vi "Facade.vi"(0 "Data In":T4, 2 "Display State In":T2, 3 "Container State":T3) -> (6 "Data Out":T4, 7 "Display State Out":T2, 8 "Action":T1)   [LabVIEW 2017, in "XListGraph.lvlib" / "XListGraph.xctl"]
uses:
  XListGraph.xctl
  Data.ctl
  <vilib>/_xctls/Container State.ctl
  State.ctl
  Support/def-XListGraphOper.ctl
  <vilib>/_xctls/Action.ctl
  <userlib>/_OpenG.lib/array/array.llb/Index 1D Array Elements (String)__ogtk.vi
  <userlib>/_OpenG.lib/array/array.llb/Filter 1D Array (String)__ogtk.vi
  <userlib>/_OpenG.lib/string/string.llb/Trim Whitespace (String Array)__ogtk.vi
  <userlib>/_OpenG.lib/array/array.llb/Filter 1D Array with Scalar (I32)__ogtk.vi
  <userlib>/_OpenG.lib/array/array.llb/Filter 1D Array (I32)__ogtk.vi
  <userlib>/_OpenG.lib/array/array.llb/Remove Duplicates from 1D Array (I32)__ogtk.vi
  <userlib>/_OpenG.lib/array/array.llb/Sort 1D Array (I32)__ogtk.vi
  <userlib>/_OpenG.lib/array/array.llb/Search 1D Array (String)__ogtk.vi
  <vilib>/_xctls/XControlSupport.lvlib
panel:
  in  "Listbox":i32[](listbox)
  out "Waveform Graph":waveform(dbl)[](graph)
  in  "Tab":enum32{""}(tab)
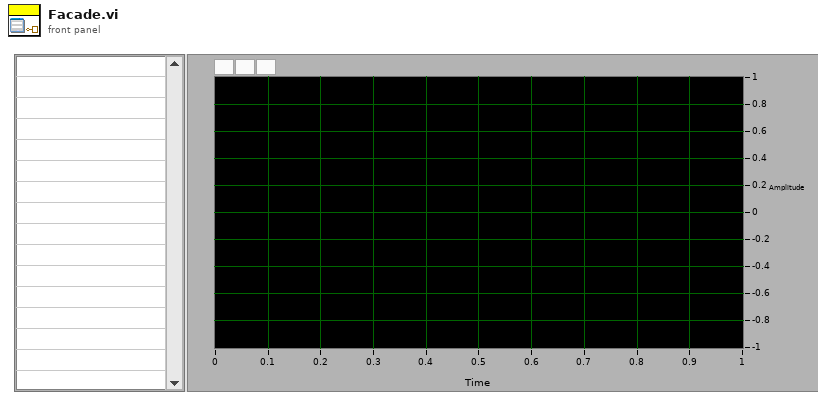
[diagram p1: front panel]
types:
  T1 = typedef "XControlSupport.lvlib/Action.ctl" = cluster{"Data Changed?":bool, "State Changed?":bool, "Action Name":string}
  T2 = typedef "XListGraph.lvlib/XListGraph.xctl/State.ctl" = cluster{"ListWindowSpliterPos":i32, "ListWindowSpliterLocked":bool, "axes":cluster{"X":cluster{"Label":string, "Unit":string}, "Y":cluster{"Label":string, "Unit":string}}, "Next State":string, "User Event":refnum<user-event>, "Plot Names":string[], "Visible Plot Names":string[], "Selected Plot Names":string[]}
  T3 = typedef "XControlSupport.lvlib/Container State.ctl" = cluster{"Indicator?":bool, "Run Mode?":bool, " Refnum":refnum<vi>}
  T4 = typedef "XListGraph.lvlib/XListGraph.xctl/Data.ctl" = waveform(dbl)[]
  T5 = typedef "LVPoint32TypeDef.ctl" = cluster{"Horizontal":i32, "Vertical":i32}
  T6 = typedef "LVRectTypeDef.ctl" = cluster{"Left":i16, "Top":i16, "Right":i16, "Bottom":i16}
  T7 = cluster{"Core":cluster{"Current VI Reference":refnum<vi>, "Close Panel on Exit?":bool}, "Splitter":refnum<vi>, "GraphRef":refnum<vi>, "ListboxRef":refnum<vi>, "Tab":refnum<vi>, "Active Menu Items":string[]}
  T8 = cluster{"Current VI Reference":refnum<vi>, "Close Panel on Exit?":bool}
  T9 = typedef "XListGraph.lvlib/XListGraph.xctl/def-wfProps.ctl" = cluster{"NI_ChannelName":string, "NI_ChannelUnit":string}
  T10 = typedef "XListGraph.lvlib/XListGraph.xctl/def-XListGraphOper.ctl" = u16
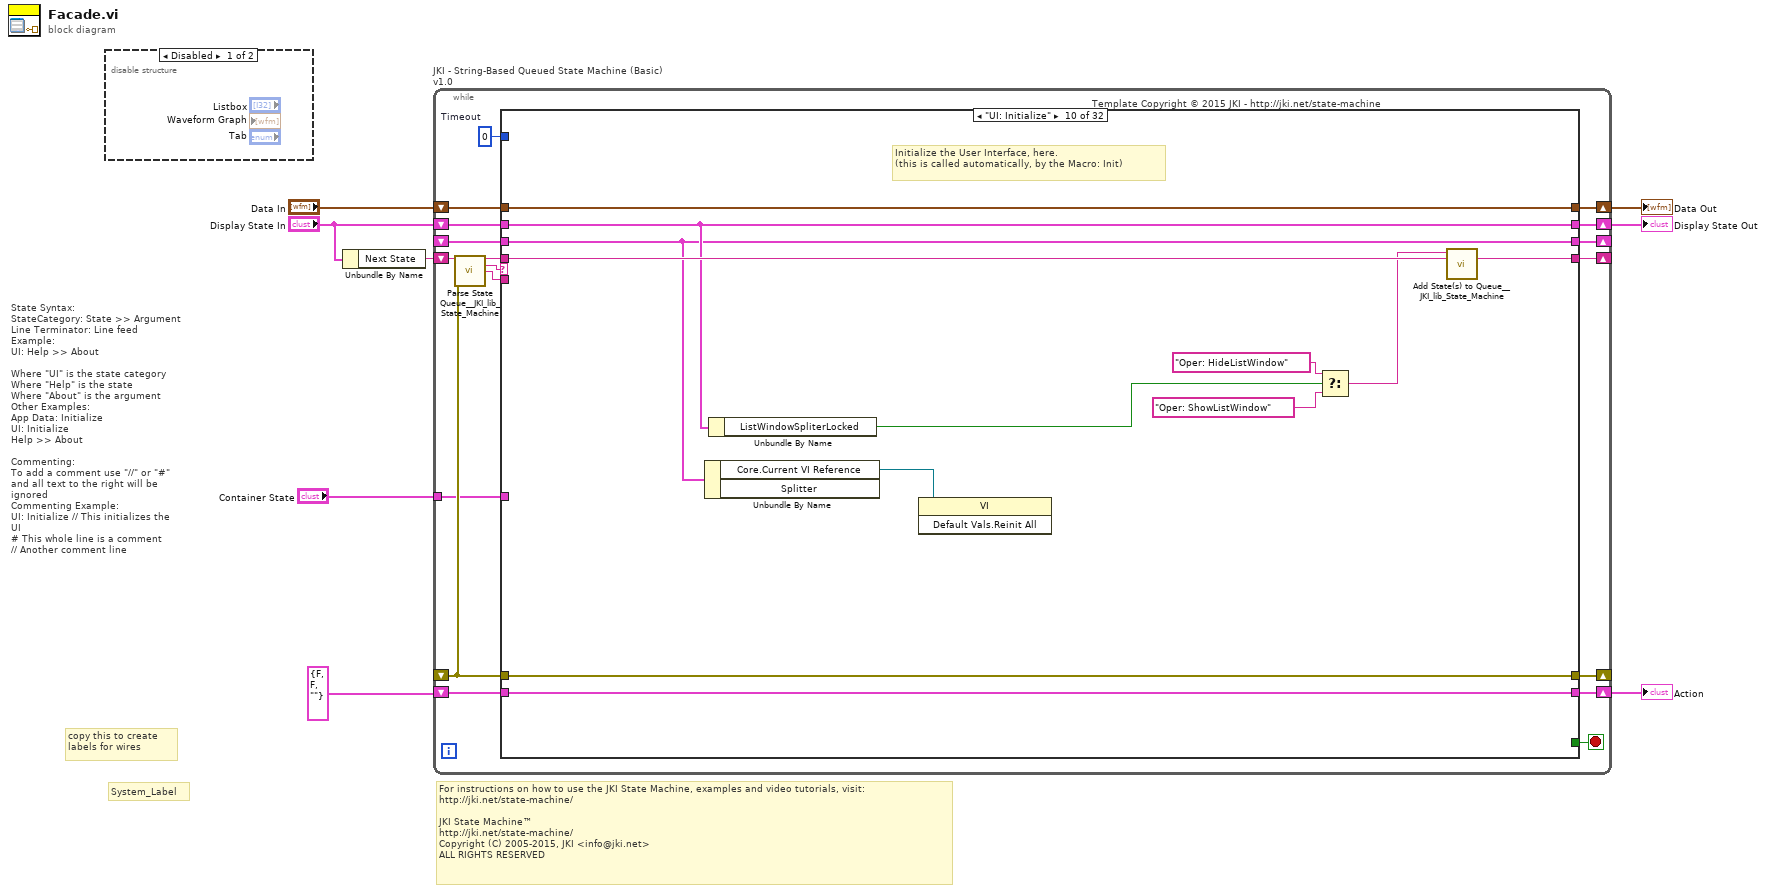
[diagram p0: block diagram]
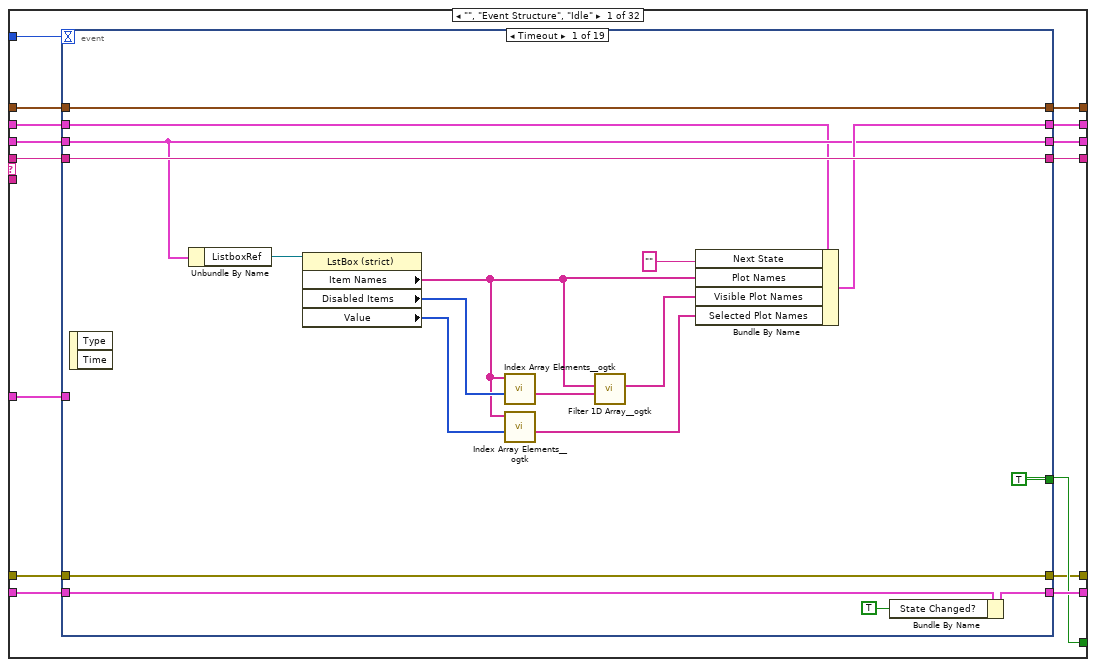
[diagram p3: hidden frame]
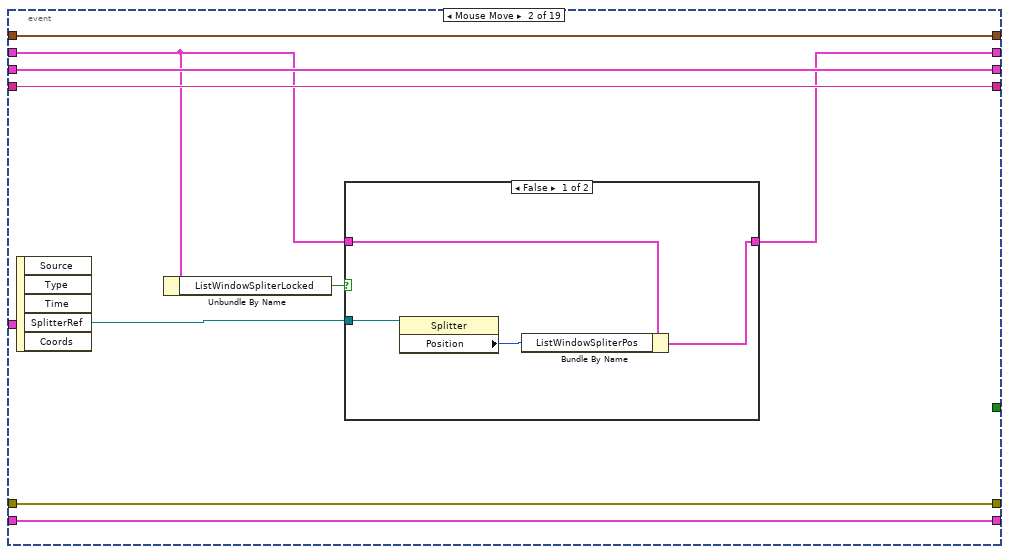
[diagram p4: hidden frame]
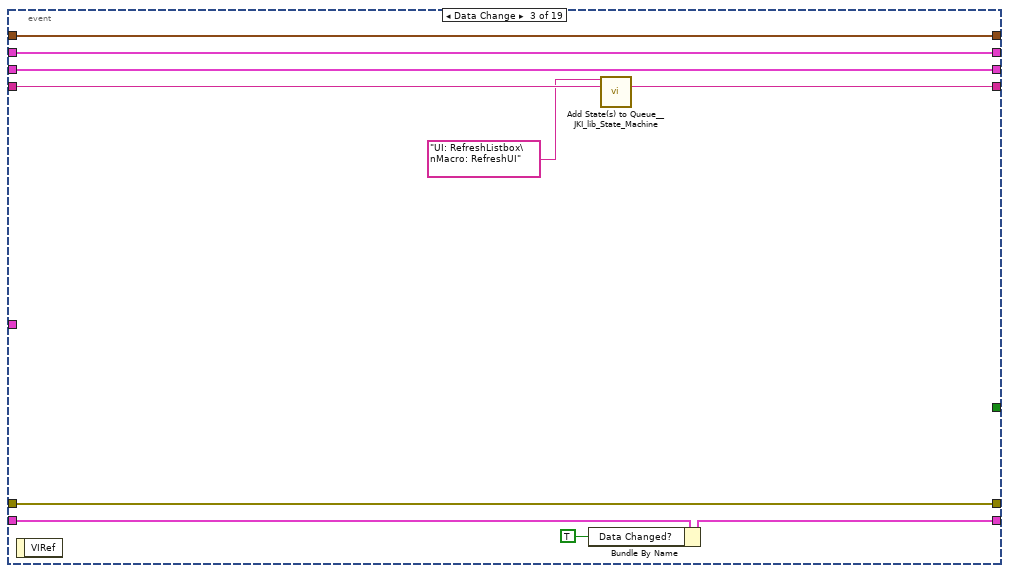
[diagram p6: hidden frame]
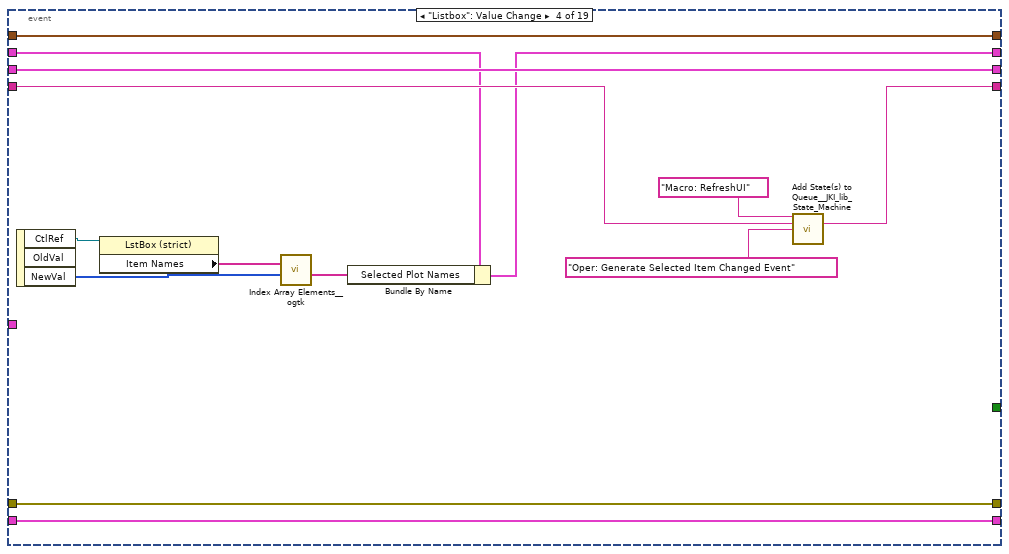
[diagram p7: hidden frame]
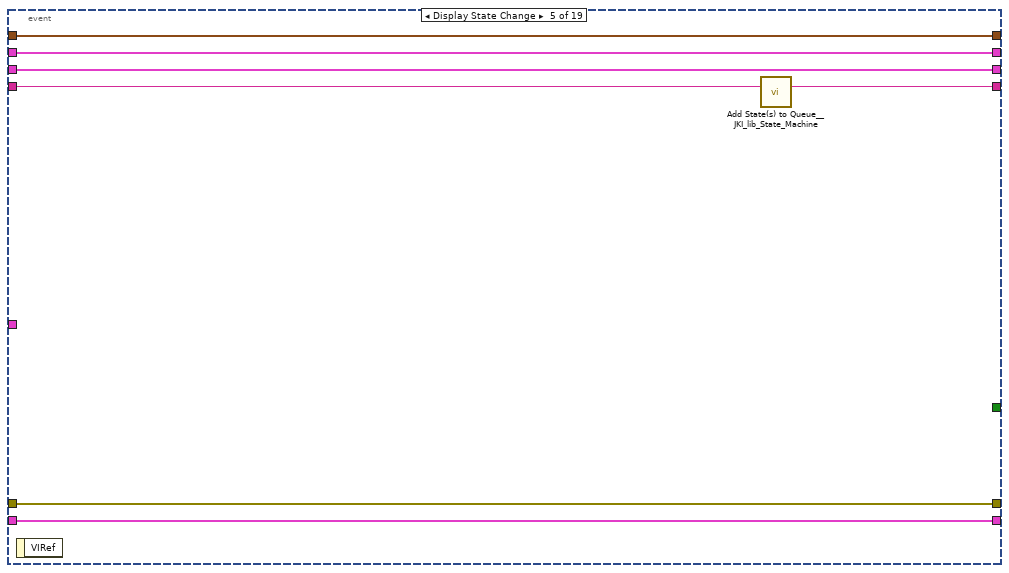
[diagram p8: hidden frame]
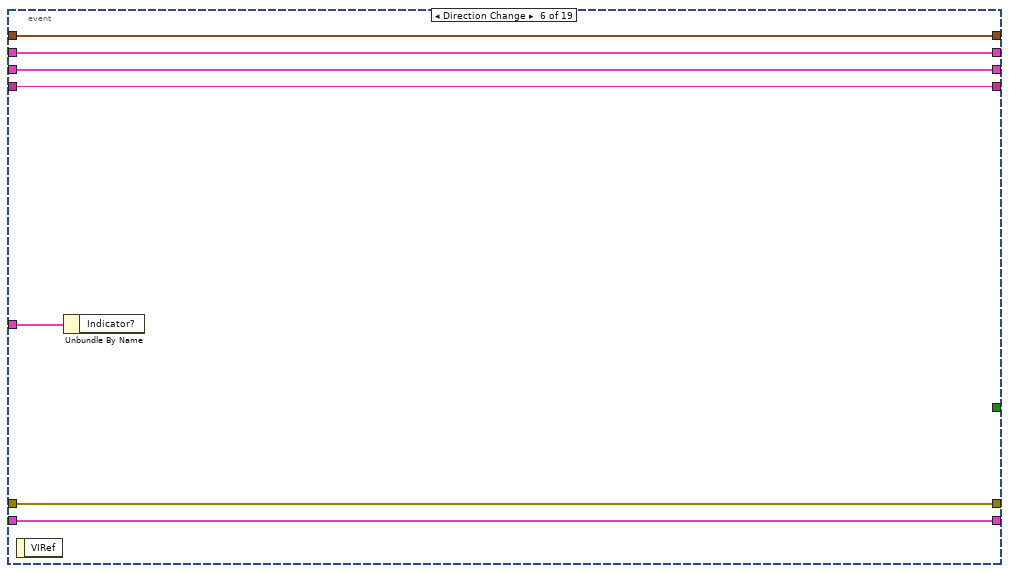
[diagram p9: hidden frame]
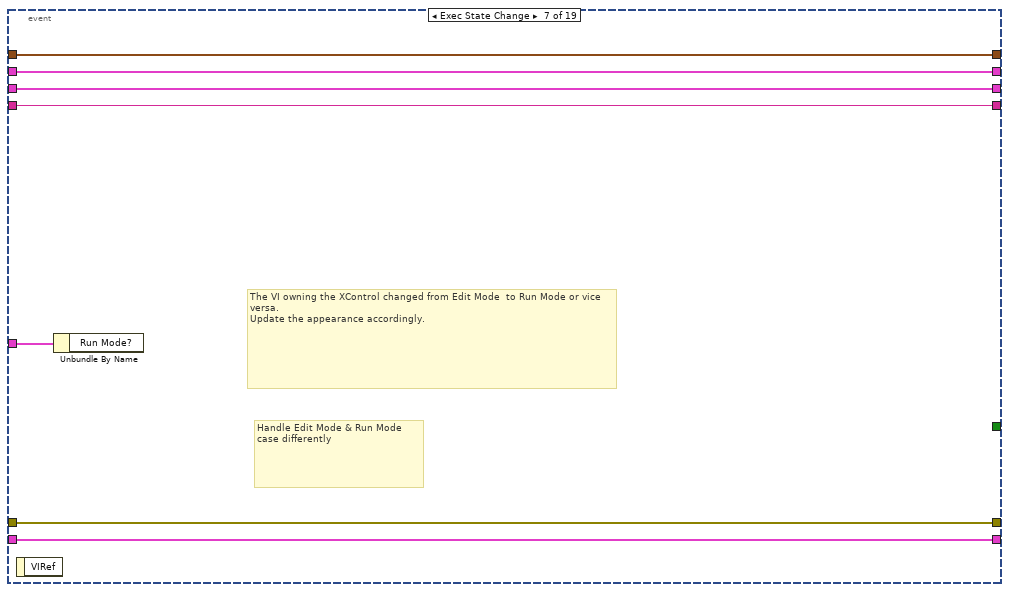
[diagram p10: hidden frame]
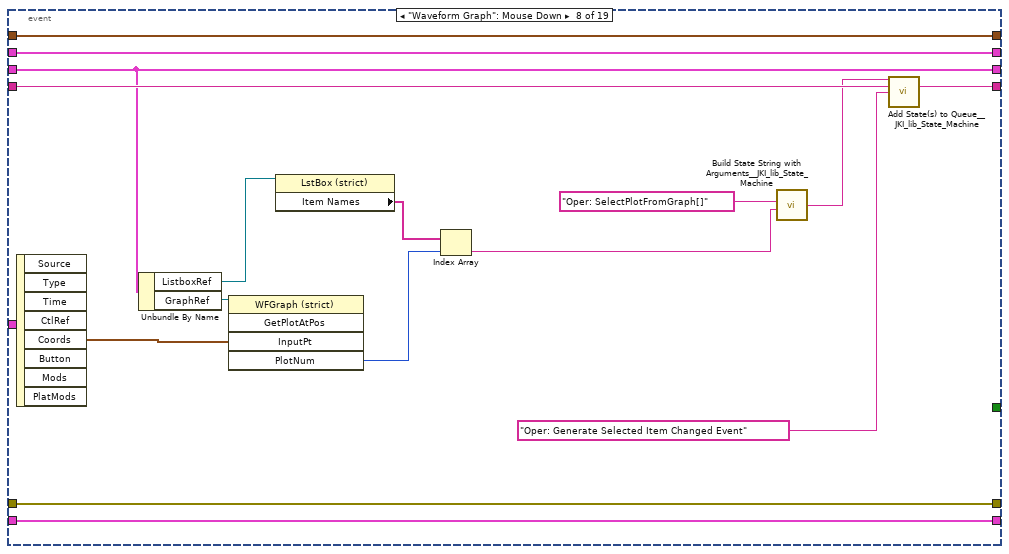
[diagram p11: hidden frame]
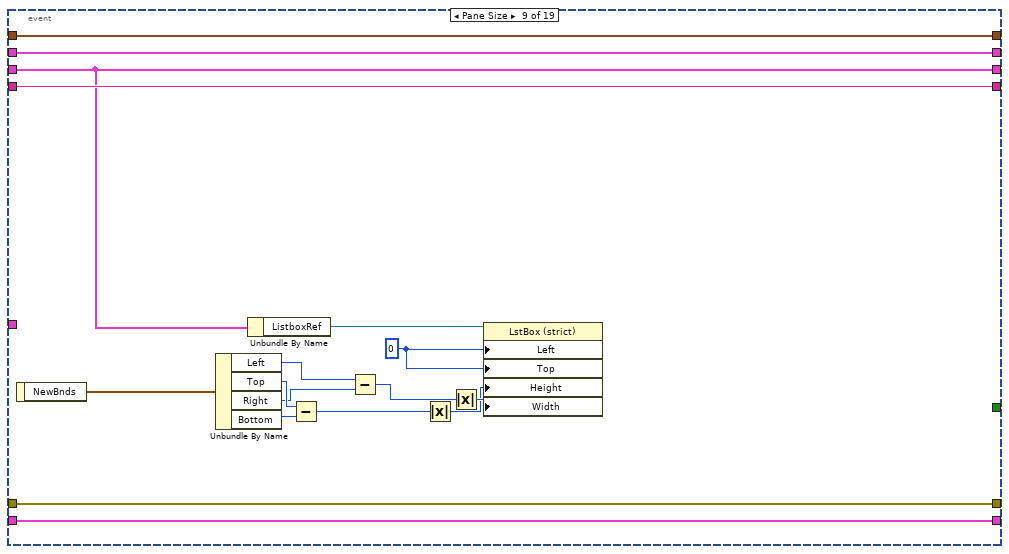
[diagram p12: hidden frame]
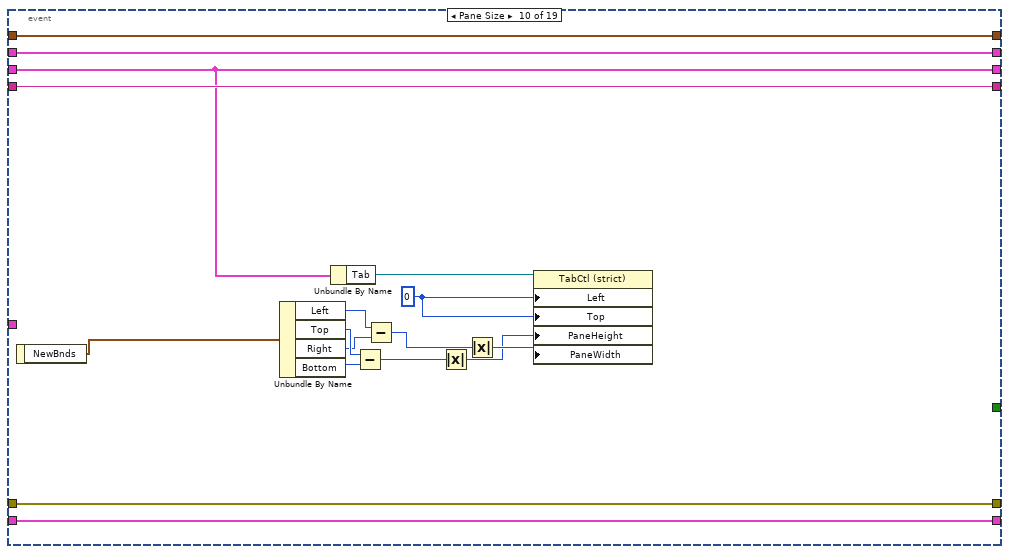
[diagram p13: hidden frame]
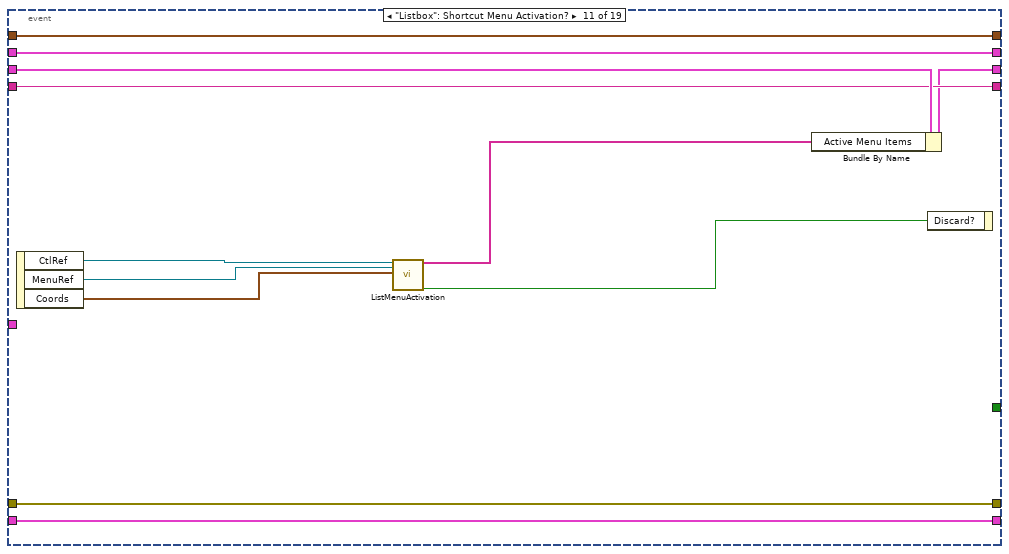
[diagram p14: hidden frame]
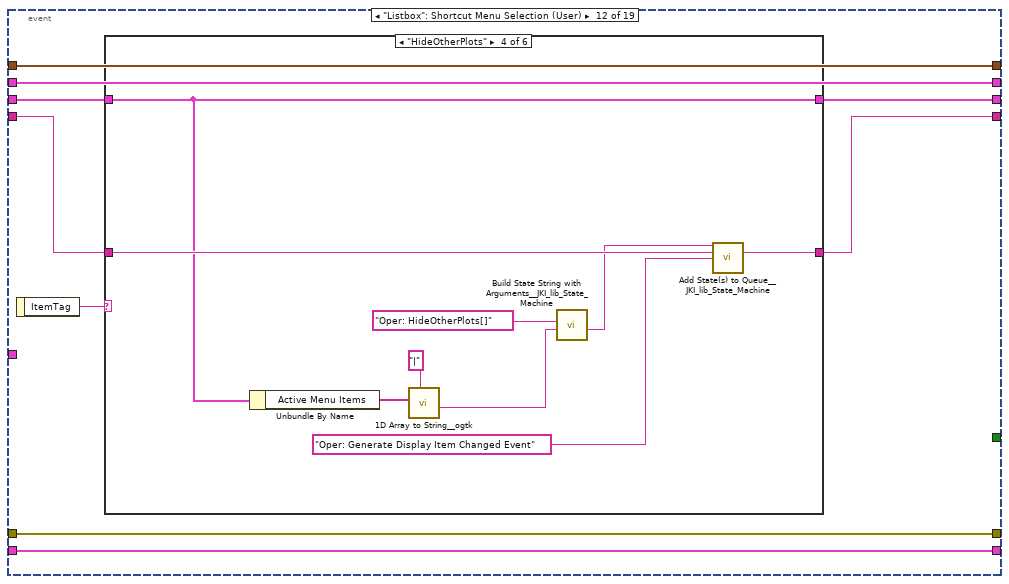
[diagram p15: hidden frame]
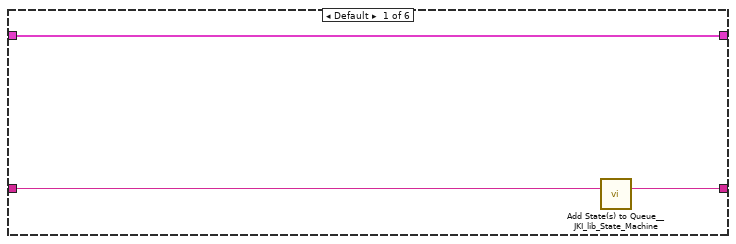
[diagram p16: hidden frame]
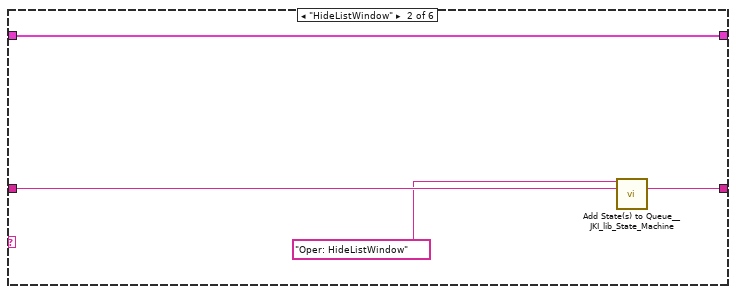
[diagram p17: hidden frame]
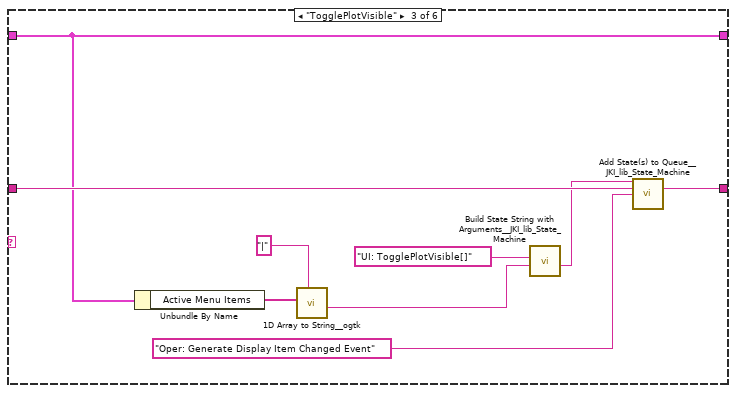
[diagram p18: hidden frame]
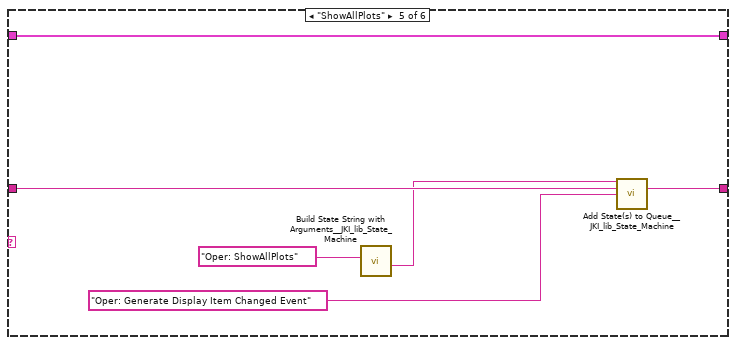
[diagram p19: hidden frame]
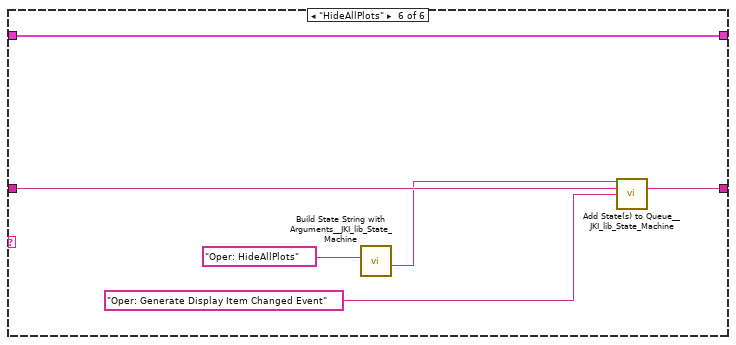
[diagram p20: hidden frame]
diagram:
  # "For instructions on how to use the JKI State Machine, examples and video tutorials, visit:\nhttp://jki.net/state-machine/\n\nJKI State Machine™\nhttp://jki.net/state-machine/\nCopyright (C) 2005-2015, JKI <info@jki.net>\nALL RIGHTS RESERVED"
  # "State Syntax:\nStateCategory: State >> Argument\nLine Terminator: Line feed\nExample:\nUI: Help >> About\n\nWhere \"UI\" is the state category\nWhere \"Help\" is the state\nWhere \"About\" is the argument\nOther Examples:\nApp Data: Initialize\nUI: Initialize\nHelp >> About\n\nCommenting:\nTo add a comment use \"//\" or \"#\" and all text to the right will be ignored\nCommenting Example:\nUI: Initialize // This initializes the UI\n# This whole line is a comment\n// Another comment line"
  # "copy this to create labels for wires"
  # "System_Label"
  n1 = disable-structure shown="Disabled" {
    frame Disabled {
    }
    frame Enabled {
    }
  }
  n2 = Unbundle By Name("Display State In") -> ("Next State"=w1:string)
  n3 = while "JKI - String-Based Queued State Machine (Basic) v1.0" {
    shift-right: [w19] -> _
    shift-left: _ -> [w18]
    shift-right: [w22] -> _
    shift-left: _ -> [w16]
    shift-right: [w21] -> _
    shift-left: w1 -> [w23]
    shift-right: [w14] -> w7
    shift-left: T1 {"Data Changed?"=FALSE, "State Changed?"=FALSE, "Action Name"=""} ("Action") -> [w15]
    shift-right: [w11] -> w4
    shift-left: "Data In" -> [w13]
    shift-right: [w10] -> w5
    shift-left: "Display State In" -> [w12]
    tunnel: "Container State" -> [w9]
    stop <- w20 stop-if-true
    w17 = 0  # Timeout
    # "Template Copyright © 2015 JKI - http://jki.net/state-machine"
    n4 = call <vilib>:"Parse State Queue__JKI_lib_State_Machine.vi"("State Queue"=w23, "Error In (no error)"=w16) -> ("Remaining States"=w25:string, "Current State"=w26:string, "Arguments"=w24:string)  [unwired: 11 in]
    n5 = case shown="\"UI: Initialize\"" w26 {
      selector: w26 -> [_ _ w304 _ _ _ _ _ _ _ _ _ _ _ _ _ _ _ _ _ _ _ _ _ _ _ _ _ _ _ _ _]
      tunnel: w25 -> [w27 w300 w308 w323 w332 w339 w352 w361 w368 w380 w389 w398 w411 w451 w467 w487 w510 w518 w526 w533 w538 w550 w569 w589 w605 w625 w635 w667 w677 w687 w699 w707]
      tunnel: w24 -> [_ _ _ _ _ _ _ _ _ _ w384 _ _ _ _ w476 _ _ _ _ _ _ w567 w587 w603 w623 w634 w655 _ _ _ _]
      tunnel: w18 -> [w29 w297 w306 w319 w329 w336 _ w356 w365 w374 w387 w394 w403 w426 w461 w481 w507 w515 w523 w530 w534 w544 w565 w586 w602 w622 w643 w654 w674 w681 w694 w702]
      tunnel: [w32 w298 w310 w320 errorcluster {"status"=FALSE, "code"=0, "source"=""} ("error out") w337 w349 w357 w366 w378 w385 w397 w412 w452 w466 w492 w508 w516 w524 w531 w543 w555 w574 w594 w610 w630 w651 w665 w678 w688 w700 w708] -> w22
      tunnel: w16 -> [w31 w298 w309 w320 w328 w337 w349 w358 w366 w378 w386 w397 w412 w452 w466 w492 w508 w516 w524 w531 w543 w555 w574 w594 w610 w630 w651 w665 w678 w688 w700 w708]
      tunnel: [w28 w299 w307 w322 w331 w338 w351 w360 w367 w379 w388 w398 w411 w451 w467 w488 w509 w517 w525 w532 w539 w551 w570 w590 w606 w626 w647 w666 w677 w687 w699 w707] -> w21
      tunnel: [w33 _ _ _ _ _ _ _ _ _ _ _ _ _ _ _ _ _ _ _ _ _ _ _ _ _ _ _ _ _ _ _] -> w20
      tunnel: [w30 w297 w306 w321 w329 w336 w350 w356 w365 w374 w387 w394 w403 w426 w461 w481 w507 w515 w523 w530 w534 w544 w565 w586 w602 w622 w643 w654 w674 w681 w694 w702] -> w19
      tunnel: w17 -> [w41 _ _ _ _ _ _ _ _ _ _ _ _ _ _ _ _ _ _ _ _ _ _ _ _ _ _ _ _ _ _ _]
      tunnel: w15 -> [w38 w296 w303 w317 w326 w335 w347 w355 w364 w377 w383 w400 w410 w450 w469 w491 w506 w513 w521 w529 w542 w554 w573 w593 w609 w629 w650 w664 w676 w686 w698 w706]
      tunnel: [w37 w296 w303 w317 w326 w335 w347 w355 w364 w377 w383 w400 w410 w450 w469 w491 w506 w513 w521 w529 w542 w554 w573 w593 w609 w629 w650 w664 w676 w686 w698 w706] -> w14
      tunnel: w13 -> [w40 w295 w302 w316 w325 w334 w346 w354 w363 w376 w382 w395 w408 w438 w463 w490 w505 w512 w520 w528 w541 w553 w572 w592 w608 w628 w649 w663 w675 w685 w697 w705]
      tunnel: w12 -> [w36 w294 w301 w315 w324 w333 w345 w353 w362 w375 w381 w399 w402 w447 w468 w489 w504 w511 w519 w527 w540 w552 w571 w591 w607 w627 w648 w662 w673 w684 w693 w701]
      tunnel: [w39 w295 w302 w316 w325 w334 w346 w354 w363 w376 w382 w395 w408 w438 w463 w490 w505 w512 w520 w528 w541 w553 w572 w592 w608 w628 w649 w663 w675 w685 w697 w705] -> w11
      tunnel: [w35 w294 w301 w315 w324 w333 w345 w353 w362 w375 w381 w399 w402 w447 w468 w489 w504 w511 w519 w527 w540 w552 w571 w591 w607 w627 w648 w662 w669 w683 w693 w701] -> w10
      tunnel: w9 -> [w34 _ _ _ _ _ _ _ _ _ _ _ _ _ _ _ _ _ _ _ _ _ _ _ _ _ _ _ _ _ _ _]
      frame "", "Event Structure", "Idle" {
        n6 = event shown="[0] Timeout" {
          selector: _ -> [_ _ _ _ _ _ _ _ _ _ _ _ _ _ _ _ _ _ _]
          dyn-events: _ -> [_ _ _ _ _ _ _ _ _ _ _ _ _ _ _ _ _ _ _]
          timeout: w41 -> [_ _ _ _ _ _ _ _ _ _ _ _ _ _ _ _ _ _ _]
          tunnel: w36 -> [w42 w61 w83 w85 w98 w110 w117 w134 w151 w168 w180 w189 w232 w239 w246 w248 w261 w276 w293]
          tunnel: [w54 w62 w83 w84 w98 w110 w117 w134 w151 w168 w180 w189 w232 w239 w246 w248 w261 w276 w293] -> w35
          tunnel: [TRUE _ _ _ _ _ _ _ _ _ _ _ _ _ _ _ _ _ _] -> w33
          tunnel: w34 -> [_ _ _ _ _ w111 w118 _ _ _ _ _ _ _ _ _ _ _ _]
          tunnel: w40 -> [w57 w68 w77 w95 w104 w109 w116 w133 w150 w167 w179 w188 w231 w238 w245 w253 w260 w275 w292]
          tunnel: [w57 w68 w77 w95 w104 w109 w116 w133 w150 w167 w179 w188 w231 w238 w245 w253 w260 w275 w292] -> w39
          tunnel: [w52 w67 w81 w97 w103 w108 w115 w132 w149 w166 w178 w187 w230 w237 w244 w252 w259 w274 w291] -> w37
          tunnel: w38 -> [w58 w67 w82 w97 w103 w108 w115 w132 w149 w166 w178 w187 w230 w237 w244 w252 w259 w274 w291]
          tunnel: [w56 w66 w79 w96 w102 w107 w114 w131 w137 w165 w174 w185 w229 w236 w243 w251 w258 w273 w290] -> w32
          tunnel: w31 -> [w56 w66 w79 w96 w102 w107 w114 w131 w137 w165 w174 w185 w229 w236 w243 w251 w258 w273 w290]
          tunnel: [w50 w65 w78 w91 w101 w106 w113 w126 w135 w152 w175 w182 w228 w235 w242 w250 w257 w272 w289] -> w30
          tunnel: w29 -> [w50 w65 w78 w91 w101 w106 w113 w126 w135 w152 w177 w181 w228 w235 w242 w250 w257 w272 w289]
          tunnel: [w55 w64 w76 w94 w100 w105 w112 w128 w136 w164 w176 w183 w227 w234 w241 w249 w254 w271 w285] -> w28
          tunnel: w27 -> [w55 w64 w75 w93 w99 w105 w112 w127 w136 w164 w176 w184 w227 w234 w241 w249 w255 w271 w284]
          event Timeout {
            n7 = event-data() -> ()  [unwired: 1 in, 2 out]
            n8 = Unbundle By Name(w50) -> ("ListboxRef"=w49:refnum<vi>)
            n9 = property class="LstBox (strict)"(reference=w49) -> ("Item Names"=w45:string[], "Disabled Items"=w48:i32[], "Value"=w44:i32[])  [unwired: 1 in, 2 out]
            n10 = call-poly <userlib>:"Index Array Elements__ogtk.vi"("indices"=w48, "array"=w45) -> ("elements"=w47:string[])  [unwired: 9 in]
            n11 = call-poly <userlib>:"Index Array Elements__ogtk.vi"("indices"=w44, "array"=w45) -> ("elements"=w43:string[])  [unwired: 9 in]
            n12 = call-poly <userlib>:"Filter 1D Array__ogtk.vi"("items to filter"=w47, "array"=w45) -> ("filtered array"=w46:string[])  [unwired: 4 in, 1 out]
            n13 = Bundle By Name(cluster=w42, "Next State"="", "Plot Names"=w45, "Visible Plot Names"=w46, "Selected Plot Names"=w43) -> (w54:T2)
            n14 = Bundle By Name(cluster=w58, "State Changed?"=TRUE) -> (w52:T1)
          }
          event Mouse Move {
            n15 = event-data() -> ("SplitterRef"=w63:refnum<vi>)  [unwired: 1 in, 4 out]
            n16 = Unbundle By Name(w61) -> ("ListWindowSpliterLocked"=w60:bool)
            n17 = case shown="False" w60 {
              tunnel: w63 -> [w72 _]
              tunnel: [w71 w73] -> w62
              tunnel: w61 -> [w69 w73]
              frame False {
                n18 = property class="Splitter"(reference=w72) -> ("Position"=w70:i32)  [unwired: 1 in, 2 out]
                n19 = Bundle By Name(cluster=w69, "ListWindowSpliterPos"=w70) -> (w71:T2)
              }
              frame True {
              }
            }
          }
          event Data Change {
            n20 = event-data() -> ()  [unwired: 1 in, 1 out]
            n21 = Bundle By Name(cluster=w82, "Data Changed?"=TRUE) -> (w81:T1)
            n22 = call <vilib>:"Add State(s) to Queue__JKI_lib_State_Machine.vi"("State(s) in Front (\"\")"="UI: RefreshListbox\nMacro: RefreshUI" ("State(s) in Front (\"\")"), "State(s) in (\"\")"=w75) -> ("States Out"=w76:string)  [unwired: 13 in]
          }
          event "Listbox": Value Change {
            n23 = event-data() -> ("CtlRef"=w88:refnum<vi>, "NewVal"=w89:i32[])  [unwired: 1 in, 1 out]
            n24 = property class="LstBox (strict)"(reference=w88) -> ("Item Names"=w87:string[])  [unwired: 1 in, 2 out]
            n25 = call-poly <userlib>:"Index Array Elements__ogtk.vi"("indices"=w89, "array"=w87) -> ("elements"=w86:string[])  [unwired: 9 in]
            n26 = Bundle By Name(cluster=w85, "Selected Plot Names"=w86) -> (w84:T2)
            n27 = call <vilib>:"Add State(s) to Queue__JKI_lib_State_Machine.vi"("State(s) in Front (\"\")"="Macro: RefreshUI" ("State(s) in Front (\"\")"), "State(s) in (\"\")"=w93, "State(s) at Back (\"\")"="Oper: Generate Selected Item Changed Event" ("State(s) at Back (\"\")")) -> ("States Out"=w94:string)  [unwired: 12 in]
          }
          event Display State Change {
            n28 = event-data() -> ()  [unwired: 1 in, 1 out]
            n29 = call <vilib>:"Add State(s) to Queue__JKI_lib_State_Machine.vi"("State(s) in (\"\")"=w99) -> ("States Out"=w100:string)  [unwired: 14 in]
          }
          event Direction Change {
            n30 = event-data() -> ()  [unwired: 1 in, 1 out]
            n31 = Unbundle By Name(w111) -> ()  [unwired: 1 out]
          }
          event Exec State Change {
            # "The VI owning the XControl changed from Edit Mode  to Run Mode or vice versa.\nUpdate the appearance accordingly."
            # "Handle Edit Mode & Run Mode\ncase differently"
            n32 = event-data() -> ()  [unwired: 1 in, 1 out]
            n33 = Unbundle By Name(w118) -> ()  [unwired: 1 out]
          }
          event "Waveform Graph": Mouse Down {
            n34 = event-data() -> ("Coords"=w129:T5)  [unwired: 1 in, 7 out]
            n35 = Unbundle By Name(w126) -> ("ListboxRef"=w120:refnum<vi>, "GraphRef"=w130:refnum<vi>)
            n36 = invoke class="WFGraph (strict)" method="GetPlotAtPos"(reference=w130, "InputPt"=w129) -> ("PlotNum"=w119:i32)  [unwired: 3 in, 4 out]
            n37 = property class="LstBox (strict)"(reference=w120) -> ("Item Names"=w122:string[])  [unwired: 1 in, 2 out]
            n38 = Index Array(array=w122, index=w119) -> (element=w121:string)
            n39 = call <vilib>:"Build State String with Arguments__JKI_lib_State_Machine.vi"("Arguments (\"\")"=w121, "State"="Oper: SelectPlotFromGraph[]") -> ("State with Arguments"=w125:string)  [unwired: 4 in]
            n40 = call <vilib>:"Add State(s) to Queue__JKI_lib_State_Machine.vi"("State(s) in Front (\"\")"=w125, "State(s) in (\"\")"=w127, "State(s) at Back (\"\")"="Oper: Generate Selected Item Changed Event" ("State")) -> ("States Out"=w128:string)  [unwired: 12 in]
          }
          event Pane Size {
            w147 = 0 ("Position:Left")
            n41 = event-data() -> ("NewBnds"=w146:T6)  [unwired: 1 in]
            n42 = Unbundle By Name(w146) -> ("Left"=w141:i16, "Top"=w144:i16, "Right"=w142:i16, "Bottom"=w145:i16)
            n43 = Unbundle By Name(w135) -> ("ListboxRef"=w148:refnum<vi>)
            n44 = Subtract(x=w144, y=w145) -> (x-y=w143:i16)
            n45 = Subtract(x=w141, y=w142) -> (x-y=w140:i16)
            n46 = Absolute Value(x=w143) -> (abs(x)=w138:i16)
            n47 = Absolute Value(x=w140) -> (abs(x)=w139:i16)
            n48 = property class="LstBox (strict)"(reference=w148, "Left"=w147, "Top"=w147, "Height"=w138, "Width"=w139) -> ()  [unwired: 1 in, 2 out]
          }
          event Pane Size {
            w162 = 0 ("Position:Left")
            n49 = event-data() -> ("NewBnds"=w153:T6)  [unwired: 1 in]
            n50 = Unbundle By Name(w153) -> ("Left"=w157:i16, "Top"=w160:i16, "Right"=w158:i16, "Bottom"=w161:i16)
            n51 = Unbundle By Name(w152) -> ("Tab"=w163:refnum<vi>)
            n52 = Subtract(x=w160, y=w161) -> (x-y=w159:i16)
            n53 = Subtract(x=w157, y=w158) -> (x-y=w156:i16)
            n54 = Absolute Value(x=w159) -> (abs(x)=w154:i16)
            n55 = Absolute Value(x=w156) -> (abs(x)=w155:i16)
            n56 = property class="TabCtl (strict)"(reference=w163, "Left"=w162, "Top"=w162, "PaneHeight"=w154, "PaneWidth"=w155) -> ()  [unwired: 1 in, 2 out]
          }
          event "Listbox": Shortcut Menu Activation? {
            n57 = event-data() -> ("CtlRef"=w173:refnum<vi>, "MenuRef"=w172:refnum<k9>, "Coords"=w169:T5)  [unwired: 1 in]
            n58 = call "ListMenuActivation.vi"("ListBox in"=w173, "MenuRef"=w172, "Point"=w169) -> ("Menu Items"=w171:string[], "Discard Event?"=w170:bool)  [unwired: 15 in]
            n59 = Bundle By Name(cluster=w177, "Active Menu Items"=w171) -> (w175:T7)
            n60 = event-data("Discard?"=w170) -> ()  [unwired: 1 in, 1 out]
          }
          event "Listbox": Shortcut Menu Selection (User) {
            n61 = event-data() -> ("ItemTag"=w186:string)  [unwired: 1 in]
            n62 = case shown="\"HideOtherPlots\"" w186 {
              tunnel: [w192 w196 w205 w214 w220 w226] -> w183
              tunnel: w184 -> [w191 w195 w204 w213 w219 w225]
              tunnel: [w190 w193 w200 w209 w216 w222] -> w182
              tunnel: w181 -> [w190 w193 w200 w209 w216 w222]
              frame Default {
                n63 = call <vilib>:"Add State(s) to Queue__JKI_lib_State_Machine.vi"("State(s) in (\"\")"=w191) -> ("States Out"=w192:string)  [unwired: 14 in]
              }
              frame "HideListWindow" {
                n64 = call <vilib>:"Add State(s) to Queue__JKI_lib_State_Machine.vi"("State(s) in Front (\"\")"="Oper: HideListWindow" ("State(s) in Front (\"\")"), "State(s) in (\"\")"=w195) -> ("States Out"=w196:string)  [unwired: 13 in]
              }
              frame "TogglePlotVisible" {
                n65 = Unbundle By Name(w200) -> ("Active Menu Items"=w199:string[])
                n66 = call <userlib>:"1D Array to String__ogtk.vi"("delimiter (Tab)"="|", "Array of Strings"=w199) -> ("delimited string"=w197:string)  [unwired: 9 in]
                n67 = call <vilib>:"Build State String with Arguments__JKI_lib_State_Machine.vi"("Arguments (\"\")"=w197, "State"="UI: TogglePlotVisible[]" ("State(s) in Front (\"\")")) -> ("State with Arguments"=w203:string)  [unwired: 4 in]
                n68 = call <vilib>:"Add State(s) to Queue__JKI_lib_State_Machine.vi"("State(s) in Front (\"\")"=w203, "State(s) in (\"\")"=w204, "State(s) at Back (\"\")"="Oper: Generate Display Item Changed Event" ("State(s) in Front (\"\")")) -> ("States Out"=w205:string)  [unwired: 12 in]
              }
              frame "HideOtherPlots" {
                n69 = Unbundle By Name(w209) -> ("Active Menu Items"=w207:string[])
                n70 = call <userlib>:"1D Array to String__ogtk.vi"("delimiter (Tab)"="|", "Array of Strings"=w207) -> ("delimited string"=w210:string)  [unwired: 9 in]
                n71 = call <vilib>:"Build State String with Arguments__JKI_lib_State_Machine.vi"("Arguments (\"\")"=w210, "State"="Oper: HideOtherPlots[]" ("State(s) in Front (\"\")")) -> ("State with Arguments"=w212:string)  [unwired: 4 in]
                n72 = call <vilib>:"Add State(s) to Queue__JKI_lib_State_Machine.vi"("State(s) in Front (\"\")"=w212, "State(s) in (\"\")"=w213, "State(s) at Back (\"\")"="Oper: Generate Display Item Changed Event" ("State(s) in Front (\"\")")) -> ("States Out"=w214:string)  [unwired: 12 in]
              }
              frame "ShowAllPlots" {
                n73 = call <vilib>:"Build State String with Arguments__JKI_lib_State_Machine.vi"("State"="Oper: ShowAllPlots" ("State(s) in Front (\"\")")) -> ("State with Arguments"=w218:string)  [unwired: 5 in]
                n74 = call <vilib>:"Add State(s) to Queue__JKI_lib_State_Machine.vi"("State(s) in Front (\"\")"=w218, "State(s) in (\"\")"=w219, "State(s) at Back (\"\")"="Oper: Generate Display Item Changed Event" ("State(s) in Front (\"\")")) -> ("States Out"=w220:string)  [unwired: 12 in]
              }
              frame "HideAllPlots" {
                n75 = call <vilib>:"Build State String with Arguments__JKI_lib_State_Machine.vi"("State"="Oper: HideAllPlots" ("State(s) in Front (\"\")")) -> ("State with Arguments"=w224:string)  [unwired: 5 in]
                n76 = call <vilib>:"Add State(s) to Queue__JKI_lib_State_Machine.vi"("State(s) in Front (\"\")"=w224, "State(s) in (\"\")"=w225, "State(s) at Back (\"\")"="Oper: Generate Display Item Changed Event" ("State(s) in Front (\"\")")) -> ("States Out"=w226:string)  [unwired: 12 in]
              }
            }
          }
          event "Waveform Graph": Plot Attribute Change {
            n77 = event-data() -> ()  [unwired: 1 in, 8 out]
            n78 = disable-structure shown="Disabled" {
              frame Disabled {
                n79 = One Button Dialog(message="Plot Attribute Change") -> ()  [unwired: 1 in, 1 out]
              }
              frame Enabled {
              }
            }
          }
          event "Waveform Graph": Autoscale Range Change {
            n80 = event-data() -> ()  [unwired: 1 in, 8 out]
            n81 = disable-structure shown="Disabled" {
              frame Disabled {
                n82 = One Button Dialog(message="Autoscale Range Change") -> ()  [unwired: 1 in, 1 out]
              }
              frame Enabled {
              }
            }
          }
          event "Waveform Graph": Scale Range Change {
            n83 = event-data() -> ()  [unwired: 1 in, 8 out]
            n84 = disable-structure shown="Disabled" {
              frame Disabled {
                n85 = One Button Dialog(message="Scale Range Change") -> ()  [unwired: 1 in, 1 out]
              }
              frame Enabled {
              }
            }
          }
          event "Waveform Graph": Shortcut Menu Activation? {
            n86 = event-data() -> ()  [unwired: 1 in, 1 out]
            n87 = event-data() -> ()  [unwired: 2 in, 1 out]
          }
          event "Waveform Graph": Shortcut Menu Selection (User) {
            n88 = event-data() -> ("ItemTag"=w256:string)  [unwired: 1 in, 7 out]
            n89 = case shown="\"HideListWindow\"" w256 {
              tunnel: [w263 w266 w269] -> w254
              tunnel: w255 -> [w262 w265 w268]
              frame Default {
                n90 = call <vilib>:"Add State(s) to Queue__JKI_lib_State_Machine.vi"("State(s) in (\"\")"=w262) -> ("States Out"=w263:string)  [unwired: 14 in]
              }
              frame "HideListWindow" {
                n91 = call <vilib>:"Add State(s) to Queue__JKI_lib_State_Machine.vi"("State(s) in Front (\"\")"="Oper: HideListWindow" ("State(s) in Front (\"\")"), "State(s) in (\"\")"=w265) -> ("States Out"=w266:string)  [unwired: 13 in]
              }
              frame "ShowListWindow" {
                n92 = call <vilib>:"Add State(s) to Queue__JKI_lib_State_Machine.vi"("State(s) in Front (\"\")"="Oper: ShowListWindow" ("State(s) in Front (\"\")"), "State(s) in (\"\")"=w268) -> ("States Out"=w269:string)  [unwired: 13 in]
              }
            }
          }
          event "Waveform Graph": Shortcut Menu Selection (App) {
            n93 = event-data() -> ("ItemTag"=w270:string)  [unwired: 1 in]
            n94 = case shown="\"APP_SC_CURSOR_LEGEND\", \"APP_SC_GRAPH_PALETTE\", \"APP_SC_PLOT_LEGEND\", \"APP_SC_SCALE_LEGEND\", \"APP_SC_X_SCROLLBAR\"" w270 {
              frame Default {
              }
              frame "APP_SC_CURSOR_LEGEND", "APP_SC_GRAPH_PALETTE", "APP_SC_PLOT_LEGEND", "APP_SC_SCALE_LEGEND", "APP_SC_X_SCROLLBAR" {
                n95 = invoke on="Waveform Graph" class="WFGraph (strict)" method="FitControlToPane"() -> ()  [unwired: 3 in, 3 out]
              }
            }
          }
          event "Listbox": Double Click {
            n96 = event-data() -> ("CtlRef"=w288:refnum<vi>, "Coords"=w287:T5)  [unwired: 1 in]
            n97 = invoke class="LstBox (strict)" method="Point To Row"(reference=w288, "Point"=w287) -> (reference out=w286:refnum<vi>, error out=w281:errorcluster, "Row"=w280:i32)  [unwired: 5 in, 4 out]
            n98 = property class="LstBox (strict)"(reference=w286, error in=w281) -> ("Item Names"=w279:string[])  [unwired: 2 out]
            n99 = Index Array(array=w279, index=w280) -> (element=w277:string)
            n100 = call <vilib>:"Build State String with Arguments__JKI_lib_State_Machine.vi"("Arguments (\"\")"=w277, "State"="UI: TogglePlotVisible[]" ("State(s) in Front (\"\")")) -> ("State with Arguments"=w282:string)  [unwired: 4 in]
            n101 = call <vilib>:"Add State(s) to Queue__JKI_lib_State_Machine.vi"("State(s) in Front (\"\")"=w282, "State(s) in (\"\")"=w284, "State(s) at Back (\"\")"="Oper: Generate Display Item Changed Event" ("State(s) in Front (\"\")")) -> ("States Out"=w285:string)  [unwired: 12 in]
          }
        }
      }
      frame "---------- Core ----------" {
        # "Do not put any code in this frame.\n(it is a separator no-op)"
        n102 = call <vilib>:"Add State(s) to Queue__JKI_lib_State_Machine.vi"("State(s) in (\"\")"=w300) -> ("States Out"=w299:string)  [unwired: 14 in]
      }
      frame Default {
        w313 = 42 items=["No error", "Argument error", "Memory is full", "Out of zone", "End of file", "File already open", "Generic file I/O error", "File not found", "File permission error", "Disk is full", "Duplicate path", "Too many files open", "System feature not enabled", "Resource file not found", "Cannot add resource", "Resource not found", "Image not found", "Image memory error", "Pen does not exist", "Config type invalid", "Config token not found", "Config parse error", "Config memory error", "Bad external code format", "Bad external code offset", "External code not present", "Null window", "Destroy window error", "Null menu", "Print aborted", "Bad print record", "Print driver error", "Windows error during printing", "Memory error during printing", "Print dialog error", "Generic print error", "Invalid device refnum", "Device not found", "Device parameter error", "Device unit error", "Cannot open device", "Device call aborted", "Generic error", "Cancelled by user", "Object ID too low", "Object ID too high", "Object not in heap", "Unknown heap", "Unknown object (invalid DefProc)", "Unknown object (DefProc not in table)", "Message out of range", "Invalid (null) method", "Unknown message", "Manager call not supported", "Bad address", "Network operation in progress", "Network operation timed out", "Connection is busy", "Network attribute not supported", "Network error", "Address in use", "System out of memory", "Connection aborted", "Connection refused", "Not connected", "Already connected", "Connection closed", "Initialization error (interapplication manager)", "Bad occurrence", "Wait on unbound occurrence handler", "Occurrence queue overflow", "Datalog type conflict", "Unused", "Unrecognized type (interapplication manager)", "Memory corrupt", "Failed to make temporary DLL", "Old CIN version", "Drag socket not found", "Failed to load drop-object", "Failed to register OLE object", "Failed to release OLE object", "Format specifier type mismatch", "Unknown format specifier", "Too few format specifiers", "Too many format specifiers", "Scan failed", "Newer CIN version", "Error converting to variant", "Runtime menu error", "Password tampered", "Variant attribute not found", "Incompatible variant data type", "Event data is not available", "Event Store is not present", "Occurrence is not found", "Event Queue is not created", "Event info is not available", "Refnum passed is NULL", "Error retrieving Class GUID", "Error retrieving CoClass GUID", "Error retrieving TypeLib GUID.", "Bad built application magic bytes.", "Specific driver is different from the specific driver associated with the Logical Name.", "There is no session opened to the class driver.", "Max Error", "MAX - Error with config objects", "MAX - Error loading configuration", "MAX - Group not supported"]
        # "Current State"
        # "Do not delete, rename, or modify this frame.\n(this is used to capture unhandled states and typos)"
        # "Handle mistyped state name (developer tool)"
        n103 = Format Into String(format string="Software Exception: Unhandled State \"%s\"." ("message"), error in=w309, w304) -> (resulting string=w312:string, error out=w311:errorcluster)  [unwired: 1 in]
        n104 = call <vilib>:"Error Cluster From Error Code.vi"("show call chain? (False)"=TRUE, "error in (no error)"=w311, "error message (\"\")"=w312, "error code (0)"=w313) -> ("error out"=w310:errorcluster)  [unwired: 5 in]
        n105 = call <vilib>:"Add State(s) to Queue__JKI_lib_State_Machine.vi"("State(s) in (\"\")"=w308) -> ("States Out"=w307:string)  [unwired: 14 in]
      }
      frame "Initialize Core Data" {
        # "Do not delete, rename, or modify this frame.\n(this is used to determine panel behavior on exit)"
        n106 = control-ref of="Current VI Reference"() -> (w318:refnum<vi>)
        n107 = Bundle By Name(cluster=w319, "Core.Current VI Reference"=w318) -> (w321:T7)
        n108 = call <vilib>:"Add State(s) to Queue__JKI_lib_State_Machine.vi"("State(s) in (\"\")"=w323) -> ("States Out"=w322:string)  [unwired: 14 in]
      }
      frame "Error Handler" {
        # "Unhandled Error -- Display it"
        # "Handle any errors here.\nYou can also output any states to clean-up after errors occur"
        # "Clear error"
        n109 = call <vilib>:"General Error Handler.vi"("error in (no error)"=w328) -> ()  [unwired: 10 in, 5 out]
        n110 = call <vilib>:"Add State(s) to Queue__JKI_lib_State_Machine.vi"("State(s) in Front (\"\")"="/* Post Error States", "State(s) in (\"\")"=w332) -> ("States Out"=w331:string)  [unwired: 13 in]
      }
      frame "---------- Data ----------" {
        # "Do not put any code in this frame.\n(It is a separator no-op. You can make a copy of this frame to create a new Data frame)"
        n111 = call <vilib>:"Add State(s) to Queue__JKI_lib_State_Machine.vi"("State(s) in (\"\")"=w339) -> ("States Out"=w338:string)  [unwired: 14 in]
      }
      frame "Data: Initialize" {
        w340 = string[] []  # Active Menu Items
        w348 = T8 {"Current VI Reference"=refnum, "Close Panel on Exit?"=FALSE}  # Core
        # "do not delete - used by framework"
        # "Data names and types of shift register data are defined by this bundle."
        # "Initialize the shift-register data, here.\n(data names are defined by what you wire into the bundle function)"
        n112 = control-ref of="GraphRef"() -> (w343:refnum<vi>)
        n113 = control-ref of="Tab"() -> (w341:refnum<vi>)
        n114 = control-ref of="Splitter"() -> (w344:refnum<vi>)
        n115 = control-ref of="ListboxRef"() -> (w342:refnum<vi>)
        n116 = Bundle("Core"=w348, "Splitter"=w344, "GraphRef"=w343, "ListboxRef"=w342, "Tab"=w341, "Active Menu Items"=w340) -> (w350:T7)  [unwired: 1 in]
        n117 = call <vilib>:"Add State(s) to Queue__JKI_lib_State_Machine.vi"("State(s) in (\"\")"=w352) -> ("States Out"=w351:string)  [unwired: 14 in]
      }
      frame "Data: Cleanup" {
        # "Cleanup any data and references, here.\n(this is called automatically, by the Macro: Exit)"
        n118 = Unbundle By Name(w356) -> ("Core.Current VI Reference"=w359:refnum<vi>)
        n119 = Close Reference(reference=w359, error in (no error)=w358) -> (error out=w357:errorcluster)
        n120 = call <vilib>:"Add State(s) to Queue__JKI_lib_State_Machine.vi"("State(s) in (\"\")"=w361) -> ("States Out"=w360:string)  [unwired: 14 in]
      }
      frame "---------- UI ----------" {
        # "Do not put any code in this frame.\n(It is a separator no-op. You can make a copy of this frame to create a new UI frame)"
        n121 = call <vilib>:"Add State(s) to Queue__JKI_lib_State_Machine.vi"("State(s) in (\"\")"=w368) -> ("States Out"=w367:string)  [unwired: 14 in]
      }
      frame "UI: Initialize" {
        # "Initialize the User Interface, here.\n(this is called automatically, by the Macro: Init)"
        n122 = Unbundle By Name(w374) -> ("Core.Current VI Reference"=w373:refnum<vi>)  [unwired: 1 out]
        n123 = Unbundle By Name(w375) -> ("ListWindowSpliterLocked"=w372:bool)
        n124 = invoke class="VI" method="Default Vals.Reinit All"(reference=w373) -> ()  [unwired: 2 in, 3 out]
        n125 = Select(t="Oper: HideListWindow", s=w372, f="Oper: ShowListWindow") -> (s? t:f=w370:string)
        n126 = call <vilib>:"Add State(s) to Queue__JKI_lib_State_Machine.vi"("State(s) in Front (\"\")"=w370, "State(s) in (\"\")"=w380) -> ("States Out"=w379:string)  [unwired: 13 in]
      }
      frame "UI: Cursor Set" {
        # "Argument"
        # "Set and Unset Cursor Busy.\n(Usage: \"UI: Cursor Set >> Busy|Idle\")"
        n127 = case shown="\"Idle\", Default" w384 {
          tunnel: w386 -> [w391 w393]
          tunnel: [w390 w392] -> w385
          frame "Idle", Default {
            n128 = call <vilib>:"Unset Busy.vi"("error in (no error)"=w391) -> ("error out"=w390:errorcluster)  [unwired: 10 in]
          }
          frame "Busy" {
            n129 = call <vilib>:"Set Busy.vi"("error in (no error)"=w393) -> ("error out"=w392:errorcluster)  [unwired: 9 in, 1 out]
          }
        }
        n130 = call <vilib>:"Add State(s) to Queue__JKI_lib_State_Machine.vi"("State(s) in (\"\")"=w389) -> ("States Out"=w388:string)  [unwired: 14 in]
      }
      frame "UI: UpdateWaveformGraph" {
        n131 = Unbundle By Name(w394) -> ("GraphRef"=w396:refnum<vi>)
        n132 = property class="WFGraph (strict)"(reference=w396, "Value"=w395) -> ()  [unwired: 1 in, 2 out]
      }
      frame "UI: UpdateWfProps" {
        n133 = Unbundle By Name(w403) -> ("GraphRef"=w407:refnum<vi>, "ListboxRef"=w406:refnum<vi>)
        n134 = Unbundle By Name(w402) -> ("Plot Names"=w401:string[])
        n135 = property class="LstBox (strict)"(reference=w406) -> ("Value"=w405:i32[], "Disabled Items"=w404:i32[])  [unwired: 1 in, 2 out]
        n136 = Array Size(array=w408) -> (size(s)=w409:i32)
        n137 = for {
          N: w409 -> [_]
          tunnel: w405 -> [w421]
          tunnel: w407 -> [w422]
          tunnel: w404 -> [w417]
          tunnel: w401 -> [w415]
          i -> [w414]
          n138 = Search 1D Array(1D array=w421, element=w414) -> (index of element=w420:i32)  [unwired: 1 in]
          n139 = Search 1D Array(1D array=w417, element=w414) -> (index of element=w418:i32)  [unwired: 1 in]
          n140 = Index Array(array=w415, index=w414) -> (element=w413:string)
          n141 = Less Than 0?(x=w418) -> (x < 0?=w416:bool)
          n142 = Greater Or Equal To 0?(x=w420) -> (x >= 0?=w419:bool)
          n143 = Select(t=3, s=w419, f=1) -> (s? t:f=w423:i32)
          n144 = property on="Property Node" class="WFGraph (strict)"(reference=w422, "Active Plot"=w414, "Plot.Line Width"=w423, "Plot.Visible?"=w416, "Plot.Plot Name"=w413) -> ()  [unwired: 1 in, 2 out]
        }
      }
      frame "UI: UpdateWfLabels" {
        n145 = Unbundle By Name(w426) -> ("GraphRef"=w449:refnum<vi>, "ListboxRef"=w448:refnum<vi>)
        n146 = property class="LstBox (strict)"(reference=w448) -> ("Value"=w430:i32[])  [unwired: 1 in, 2 out]
        n147 = Unbundle By Name(w447) -> ("axes.X.Label"=w446:string, "axes.X.Unit"=w443:string, "axes.Y.Label"=w433:string, "axes.Y.Unit"=w431:string)
        n148 = Array Size(array=w430) -> (size(s)=w437:i32)
        n149 = Index Array(array=w430) -> (element=w429:i32)  [unwired: 1 in]
        n150 = Greater Or Equal To 0?(x=w429) -> (x >= 0?=w427:bool)
        n151 = Equal?(x=w437, y=1) -> (x = y?=w435:bool)
        n152 = And(x=w427, y=w435) -> (x .and. y?=w428:bool)
        n153 = case shown="True" w428 {
          tunnel: w438 -> [_ w460]
          tunnel: [w454 w456] -> w434
          tunnel: w433 -> [w454 _]
          tunnel: [w453 w457] -> w432
          tunnel: w431 -> [w453 _]
          tunnel: w429 -> [_ w455]
          frame False {
          }
          frame True {
            n154 = Index Array(array=w460, index=w455) -> (element=w459:waveform(dbl))
            n155 = call "WavefromProps.vi"("signal in"=w459) -> ("Waveform Properties"=w458:T9)  [unwired: 9 in, 1 out]
            n156 = Unbundle(w458) -> ("NI_ChannelName"=w456:string, "NI_ChannelUnit"=w457:string)
          }
        }
        n157 = call "ConcatenateLabel.vi"("Unit"=w443, "Label in"=w446) -> ("Boolean"=w444:bool, "Unit (dup)"=w442:string, "Label out"=w445:string)  [unwired: 7 in]
        n158 = call "ConcatenateLabel.vi"("Unit"=w432, "Label in"=w434) -> ("Boolean"=w439:bool, "Unit (dup)"=w440:string, "Label out"=w441:string)  [unwired: 7 in]
        n159 = property on="Property Node" class="WFGraph (strict)"(reference=w449, "XScale.NameLbl.Text"=w445, "XScale.UnitLabel.Text"=w442, "XScale.UnitLabel.Visible"=w444, "YScale.NameLbl.Text"=w441, "YScale.UnitLabel.Text"=w440, "YScale.UnitLabel.Visible"=w439) -> ()  [unwired: 1 in, 2 out]
      }
      frame "UI: RefreshListbox" {
        n160 = Unbundle By Name(w461) -> ("ListboxRef"=w465:refnum<vi>)
        n161 = for {
          tunnel: w463 -> [w474] mode=indexing
          tunnel: [w473] -> _ mode=indexing
          tunnel: [w470] -> w464 mode=indexing
          n162 = Get Waveform Attribute(5:"", 6:"NI_ChannelName", 7:w474) -> (1:w470:string, 3:w473:waveform(dbl))  [unwired: 1 in, 2 out]
        }
        n163 = property class="LstBox (strict)" props=["Disabled Items"](reference=w465) -> (reference out=w462:refnum<vi>)  [unwired: 1 in, 2 out]
        n164 = property class="LstBox (strict)"(reference=w462, "Item Names"=w464) -> ()  [unwired: 1 in, 2 out]
      }
      frame "UI: TogglePlotVisible[]" {
        n165 = Unbundle By Name(w481) -> ("ListboxRef"=w485:refnum<vi>)
        n166 = call <userlib>:"String to 1D Array__ogtk.vi"("delimiter (Tab)"="|", "string"=w476) -> ("Array of Strings"=w480:string[])  [unwired: 9 in]
        n167 = property class="LstBox (strict)"(reference=w485) -> (reference out=w484:refnum<vi>, "Disabled Items"=w483:i32[], "Item Names"=w477:string[])  [unwired: 1 in, 1 out]
        n168 = call-poly <userlib>:"Trim Whitespace__ogtk.vi"("String in"=w480) -> ("String out"=w478:string[])  [unwired: 6 in]
        n169 = call-poly <userlib>:"Filter 1D Array__ogtk.vi"("items to filter"=w478, "array"=w477) -> ("filtered item indices"=w475:i32[])  [unwired: 4 in, 1 out]
        n170 = for {
          tunnel: w475 -> [w493] mode=indexing
          shift-right: [w494] -> w482
          shift-left: w483 -> [w495]
          n171 = Search 1D Array(1D array=w495, element=w493) -> (index of element=w497:i32)  [unwired: 1 in]
          n172 = Greater Or Equal To 0?(x=w497) -> (x >= 0?=w496:bool)
          n173 = case shown="True" w496 {
            tunnel: w495 -> [w500 w503]
            tunnel: w493 -> [w498 w502]
            tunnel: [w499 w501] -> w494
            frame False {
              n174 = Build Array (concatenate)(w500, w498) -> (w499:i32[])
            }
            frame True {
              n175 = call-poly <userlib>:"Filter 1D Array__ogtk.vi"("items to filter"=w502, "array"=w503) -> ("filtered array"=w501:i32[])  [unwired: 4 in, 1 out]
            }
          }
        }
        n176 = property class="LstBox (strict)"(reference=w484, "Disabled Items"=w482) -> ()  [unwired: 1 in, 2 out]
        n177 = call <vilib>:"Add State(s) to Queue__JKI_lib_State_Machine.vi"("State(s) in Front (\"\")"="UI: UpdateWfProps" ("State(s) in Front (\"\")"), "State(s) in (\"\")"=w487) -> ("States Out"=w488:string)  [unwired: 13 in]
      }
      frame "---------- Macro ----------" {
        # "Do not put any code in this frame.\n(It is a separator no-op. You can make a copy of this frame to create a new Macro frame)"
        n178 = call <vilib>:"Add State(s) to Queue__JKI_lib_State_Machine.vi"("State(s) in (\"\")"=w510) -> ("States Out"=w509:string)  [unwired: 14 in]
      }
      frame "Macro: Initialize" {
        # "Initialization Macro\n(This is called once, when the VI starts)"
        n179 = call <vilib>:"Add State(s) to Queue__JKI_lib_State_Machine.vi"("State(s) in Front (\"\")"="Data: Initialize\nInitialize Core Data\nUI: Initialize", "State(s) in (\"\")"=w518) -> ("States Out"=w517:string)  [unwired: 13 in]
      }
      frame "Macro: RefreshUI" {
        n180 = call <vilib>:"Add State(s) to Queue__JKI_lib_State_Machine.vi"("State(s) in Front (\"\")"="UI: UpdateWaveformGraph\nUI: UpdateWfProps\nUI: UpdateWfLabels", "State(s) in (\"\")"=w526) -> ("States Out"=w525:string)  [unwired: 13 in]
      }
      frame "---------- Operation ----------" {
        n181 = call <vilib>:"Add State(s) to Queue__JKI_lib_State_Machine.vi"("State(s) in (\"\")"=w533) -> ("States Out"=w532:string)  [unwired: 14 in]
      }
      frame "Oper: ShowAllPlots" {
        n182 = Unbundle By Name(w534) -> ("ListboxRef"=w536:refnum<vi>)
        n183 = property class="LstBox (strict)"(reference=w536, "Disabled Items"=i32[] []) -> ()  [unwired: 1 in, 2 out]
        n184 = call <vilib>:"Add State(s) to Queue__JKI_lib_State_Machine.vi"("State(s) in Front (\"\")"="UI: UpdateWfProps" ("State(s) in Front (\"\")"), "State(s) in (\"\")"=w538) -> ("States Out"=w539:string)  [unwired: 13 in]
      }
      frame "Oper: HideAllPlots" {
        n185 = Unbundle By Name(w544) -> ("ListboxRef"=w548:refnum<vi>)
        n186 = property class="LstBox (strict)"(reference=w548) -> (reference out=w547:refnum<vi>, "Item Names"=w546:string[])  [unwired: 1 in, 1 out]
        n187 = for {
          tunnel: w546 -> [_] mode=indexing
          tunnel: [w556] -> w545 mode=indexing
          i -> [w556]
        }
        n188 = property class="LstBox (strict)"(reference=w547, "Disabled Items"=w545) -> ()  [unwired: 1 in, 2 out]
        n189 = call <vilib>:"Add State(s) to Queue__JKI_lib_State_Machine.vi"("State(s) in Front (\"\")"="UI: UpdateWfProps" ("State(s) in Front (\"\")"), "State(s) in (\"\")"=w550) -> ("States Out"=w551:string)  [unwired: 13 in]
      }
      frame "Oper: AddToVisiblePlotList[]" {
        n190 = Unbundle By Name(w565) -> ("ListboxRef"=w562:refnum<vi>)
        n191 = call <userlib>:"String to 1D Array__ogtk.vi"("delimiter (Tab)"="|", "string"=w567) -> ("Array of Strings"=w564:string[])  [unwired: 9 in]
        n192 = call-poly <userlib>:"Trim Whitespace__ogtk.vi"("String in"=w564) -> ("String out"=w559:string[])  [unwired: 6 in]
        n193 = property class="LstBox (strict)"(reference=w562) -> (reference out=w561:refnum<vi>, "Item Names"=w560:string[], "Disabled Items"=w557:i32[])  [unwired: 1 in, 1 out]
        n194 = call-poly <userlib>:"Filter 1D Array__ogtk.vi"("items to filter"=w559, "array"=w560) -> ("filtered item indices"=w558:i32[])  [unwired: 4 in, 1 out]
        n195 = call-poly <userlib>:"Filter 1D Array__ogtk.vi"("items to filter"=w558, "array"=w557) -> ("filtered array"=w566:i32[])  [unwired: 4 in, 1 out]
        n196 = property class="LstBox (strict)"(reference=w561, "Disabled Items"=w566) -> ()  [unwired: 1 in, 2 out]
        n197 = call <vilib>:"Add State(s) to Queue__JKI_lib_State_Machine.vi"("State(s) in Front (\"\")"="UI: UpdateWfProps" ("State(s) in Front (\"\")"), "State(s) in (\"\")"=w569) -> ("States Out"=w570:string)  [unwired: 13 in]
      }
      frame "Oper: RemoveFromVisiblePlotList[]" {
        n198 = Unbundle By Name(w586) -> ("ListboxRef"=w583:refnum<vi>)
        n199 = call <userlib>:"String to 1D Array__ogtk.vi"("delimiter (Tab)"="|", "string"=w587) -> ("Array of Strings"=w585:string[])  [unwired: 9 in]
        n200 = property class="LstBox (strict)"(reference=w583) -> (reference out=w582:refnum<vi>, "Item Names"=w581:string[], "Disabled Items"=w578:i32[])  [unwired: 1 in, 1 out]
        n201 = call-poly <userlib>:"Trim Whitespace__ogtk.vi"("String in"=w585) -> ("String out"=w580:string[])  [unwired: 6 in]
        n202 = call-poly <userlib>:"Filter 1D Array__ogtk.vi"("items to filter"=w580, "array"=w581) -> ("filtered item indices"=w579:i32[])  [unwired: 4 in, 1 out]
        n203 = Build Array (concatenate)(w578, w579) -> (w577:i32[])
        n204 = call-poly <userlib>:"Remove Duplicates from 1D Array__ogtk.vi"("Input Array"=w577) -> ("Output Array"=w576:i32[])  [unwired: 1 out]
        n205 = call-poly <userlib>:"Sort Array__ogtk.vi"("Array in"=w576) -> ("Sorted Array out"=w575:i32[])  [unwired: 9 in, 1 out]
        n206 = property class="LstBox (strict)"(reference=w582, "Disabled Items"=w575) -> ()  [unwired: 1 in, 2 out]
        n207 = call <vilib>:"Add State(s) to Queue__JKI_lib_State_Machine.vi"("State(s) in Front (\"\")"="UI: UpdateWfProps" ("State(s) in Front (\"\")"), "State(s) in (\"\")"=w589) -> ("States Out"=w590:string)  [unwired: 13 in]
      }
      frame "Oper: SelectPlotsByName[]" {
        n208 = Unbundle By Name(w602) -> ("ListboxRef"=w599:refnum<vi>)
        n209 = call <userlib>:"String to 1D Array__ogtk.vi"("delimiter (Tab)"="|", "string"=w603) -> ("Array of Strings"=w601:string[])  [unwired: 9 in]
        n210 = call-poly <userlib>:"Trim Whitespace__ogtk.vi"("String in"=w601) -> ("String out"=w596:string[])  [unwired: 6 in]
        n211 = property class="LstBox (strict)"(reference=w599) -> (reference out=w598:refnum<vi>, "Item Names"=w597:string[])  [unwired: 1 in, 1 out]
        n212 = for {
          tunnel: w597 -> [w613]
          tunnel: w596 -> [w612] mode=indexing
          tunnel: [w611] -> w595 mode=concatenating
          n213 = call-poly <userlib>:"Search Array__ogtk.vi"("Array"=w613, "Element Data"=w612) -> ("Indices of Elements"=w611:i32[])  [unwired: 7 in]
        }
        n214 = property class="LstBox (strict)"(reference=w598, "Value"=w595) -> ()  [unwired: 1 in, 2 out]
        n215 = call <vilib>:"Add State(s) to Queue__JKI_lib_State_Machine.vi"("State(s) in Front (\"\")"="UI: UpdateWfProps" ("State(s) in Front (\"\")"), "State(s) in (\"\")"=w605) -> ("States Out"=w606:string)  [unwired: 13 in]
      }
      frame "Oper: ShowPlotsByName[]" {
        n216 = Unbundle By Name(w622) -> ("ListboxRef"=w619:refnum<vi>)
        n217 = call <userlib>:"String to 1D Array__ogtk.vi"("delimiter (Tab)"="|", "string"=w623) -> ("Array of Strings"=w621:string[])  [unwired: 9 in]
        n218 = call-poly <userlib>:"Trim Whitespace__ogtk.vi"("String in"=w621) -> ("String out"=w617:string[])  [unwired: 6 in]
        n219 = property class="LstBox (strict)"(reference=w619) -> (reference out=w618:refnum<vi>, "Item Names"=w615:string[])  [unwired: 1 in, 1 out]
        n220 = call-poly <userlib>:"Filter 1D Array__ogtk.vi"("items to filter"=w617, "array"=w615) -> ("filtered array"=w616:string[])  [unwired: 4 in, 1 out]
        n221 = for {
          tunnel: w616 -> [w632] mode=indexing
          tunnel: w615 -> [w633]
          tunnel: [w631] -> w614 mode=indexing
          n222 = Search 1D Array(1D array=w633, element=w632) -> (index of element=w631:i32)  [unwired: 1 in]
        }
        n223 = property class="LstBox (strict)"(reference=w618, "Disabled Items"=w614) -> ()  [unwired: 1 in, 2 out]
        n224 = call <vilib>:"Add State(s) to Queue__JKI_lib_State_Machine.vi"("State(s) in Front (\"\")"="UI: UpdateWfProps" ("State(s) in Front (\"\")"), "State(s) in (\"\")"=w625) -> ("States Out"=w626:string)  [unwired: 13 in]
      }
      frame "Oper: HideOtherPlots[]" {
        n225 = Unbundle By Name(w643) -> ("ListboxRef"=w645:refnum<vi>)
        n226 = property class="LstBox (strict)"(reference=w645) -> (reference out=w644:refnum<vi>, "Item Names"=w639:string[])  [unwired: 1 in, 1 out]
        n227 = call <userlib>:"String to 1D Array__ogtk.vi"("delimiter (Tab)"="|", "string"=w634) -> ("Array of Strings"=w642:string[])  [unwired: 9 in]
        n228 = call-poly <userlib>:"Trim Whitespace__ogtk.vi"("String in"=w642) -> ("String out"=w640:string[])  [unwired: 6 in]
        n229 = for {
          tunnel: w639 -> [_] mode=indexing
          tunnel: [w652] -> w638 mode=indexing
          i -> [w652]
        }
        n230 = call-poly <userlib>:"Filter 1D Array__ogtk.vi"("items to filter"=w640, "array"=w639) -> ("filtered item indices"=w637:i32[])  [unwired: 4 in, 1 out]
        n231 = call-poly <userlib>:"Filter 1D Array__ogtk.vi"("items to filter"=w637, "array"=w638) -> ("filtered array"=w636:i32[])  [unwired: 4 in, 1 out]
        n232 = property class="LstBox (strict)"(reference=w644, "Disabled Items"=w636) -> ()  [unwired: 1 in, 2 out]
        n233 = call <vilib>:"Add State(s) to Queue__JKI_lib_State_Machine.vi"("State(s) in Front (\"\")"="UI: UpdateWfProps" ("State(s) in Front (\"\")"), "State(s) in (\"\")"=w635) -> ("States Out"=w647:string)  [unwired: 13 in]
      }
      frame "Oper: SelectPlotFromGraph[]" {
        # "Your code here.\n(You can make a copy of, or modify, this frame)"
        n234 = Unbundle By Name(w654) -> ("ListboxRef"=w660:refnum<vi>)
        n235 = call <userlib>:"String to 1D Array__ogtk.vi"("delimiter (Tab)"="|", "string"=w655) -> ("Array of Strings"=w659:string[])  [unwired: 9 in]
        n236 = Unbundle By Name(w654) -> ("ListboxRef"=w661:refnum<vi>)
        n237 = property class="LstBox (strict)"(reference=w660) -> ("Item Names"=w656:string[])  [unwired: 1 in, 2 out]
        n238 = call-poly <userlib>:"Trim Whitespace__ogtk.vi"("String in"=w659) -> ("String out"=w657:string[])  [unwired: 6 in]
        n239 = call-poly <userlib>:"Filter 1D Array__ogtk.vi"("items to filter"=w657, "array"=w656) -> ("filtered item indices"=w653:i32[])  [unwired: 4 in, 1 out]
        n240 = property class="LstBox (strict)"(reference=w661, "Val(Sgnl)"=w653) -> ()  [unwired: 1 in, 2 out]
        n241 = call <vilib>:"Add State(s) to Queue__JKI_lib_State_Machine.vi"("State(s) in (\"\")"=w667) -> ("States Out"=w666:string)  [unwired: 14 in]
      }
      frame "Oper: ShowListWindow" {
        w668 = FALSE ("Splitter Position Locked")
        n242 = Unbundle By Name(w673) -> ("ListWindowSpliterPos"=w672:i32)
        n243 = Unbundle By Name(w674) -> ("Splitter"=w671:refnum<vi>)
        n244 = property class="Splitter"(reference=w671, "Locked"=w668) -> (reference out=w670:refnum<vi>)  [unwired: 1 in, 1 out]
        n245 = property class="Splitter"(reference=w670, "Position"=w672) -> ()  [unwired: 1 in, 2 out]
        n246 = Bundle By Name(cluster=w673, "ListWindowSpliterLocked"=w668) -> (w669:T2)
      }
      frame "Oper: HideListWindow" {
        w679 = TRUE ("Splitter Position Locked")
        n247 = Unbundle By Name(w681) -> ("Splitter"=w682:refnum<vi>)
        n248 = while {
          shift-right: [w689] -> w680
          shift-left: w682 -> [w692]
          i -> [w690]
          stop <- w691 continue-if-true
          n249 = property class="Splitter"(reference=w692, "Position"=w690) -> (reference out=w689:refnum<vi>, error out=w691:errorcluster)  [unwired: 1 in]
        }
        n250 = Bundle By Name(cluster=w684, "ListWindowSpliterLocked"=w679) -> (w683:T2)
        n251 = property class="Splitter"(reference=w680, "Locked"=w679) -> ()  [unwired: 1 in, 2 out]
      }
      frame "Oper: Generate Selected Item Changed Event" {
        w695 = T10 0 items=["Selected Item Changed", "Display Item Changed"] ("event")
        n252 = Unbundle By Name(w693) -> ("User Event"=w696:refnum<user-event>)
        n253 = Generate User Event(user event=w696, event data cluster=w695) -> ()  [unwired: 2 in, 2 out]
      }
      frame "Oper: Generate Display Item Changed Event" {
        w703 = T10 1 items=["Selected Item Changed", "Display Item Changed"] ("event")
        n254 = Unbundle By Name(w701) -> ("User Event"=w704:refnum<user-event>)
        n255 = Generate User Event(user event=w704, event data cluster=w703) -> ()  [unwired: 2 in, 2 out]
      }
    }
  }
  "Display State Out" <- w5
  "Data Out" <- w4
  "Action" <- w7
